vi "pdNormalize.vi"   [LabVIEW 2011]
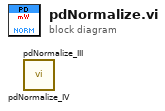
[diagram p0: block diagram]
diagram:
  n1 = call "pdNormalize_IV.vi"() -> ()  [unwired: 11 in, 5 out]
  n2 = call "pdNormalize_III.vi"() -> ()  [unwired: 12 in, 4 out]
